vi "GUI.vi"() -> ()   [LabVIEW 2019]
uses:
  <vilib>/Instr/_visa.llb/VISA Configure Serial Port (Instr).vi
panel:
  out "O":dbl
  out "T":dbl
  out "D":dbl
  out "I":dbl
  out "P":dbl
  out "F":dbl
  out "S":dbl
  in  "Stop Button":bool
  out "TS":dbl(slide) scale=0.0..255.0
  out "KD":dbl(slide) scale=0.0..10.0
  out "KI":dbl(slide) scale=0.0..0.1
  out "KP":dbl(slide) scale=0.0..10.0
  in  "COM Port":refnum<visa-resource-name>
  in  "Save Result":path
  out "Output PID":dbl(graph)
  out "Tacho Generator":dbl(knob) scale=0.0..400.0
  out "SetPoint":dbl(knob) scale=0.0..400.0
  out "Respon PID":dynamicdata(graph)
  # "ALIM SATRIA FI'I WIJAYA KUSUMA (21/483503/SV/20304)"
  # "KENDALI KECEPATAN MOTOR DC"
  # "ILHAM DWI CAHYO (21/483417/SV/20218)"
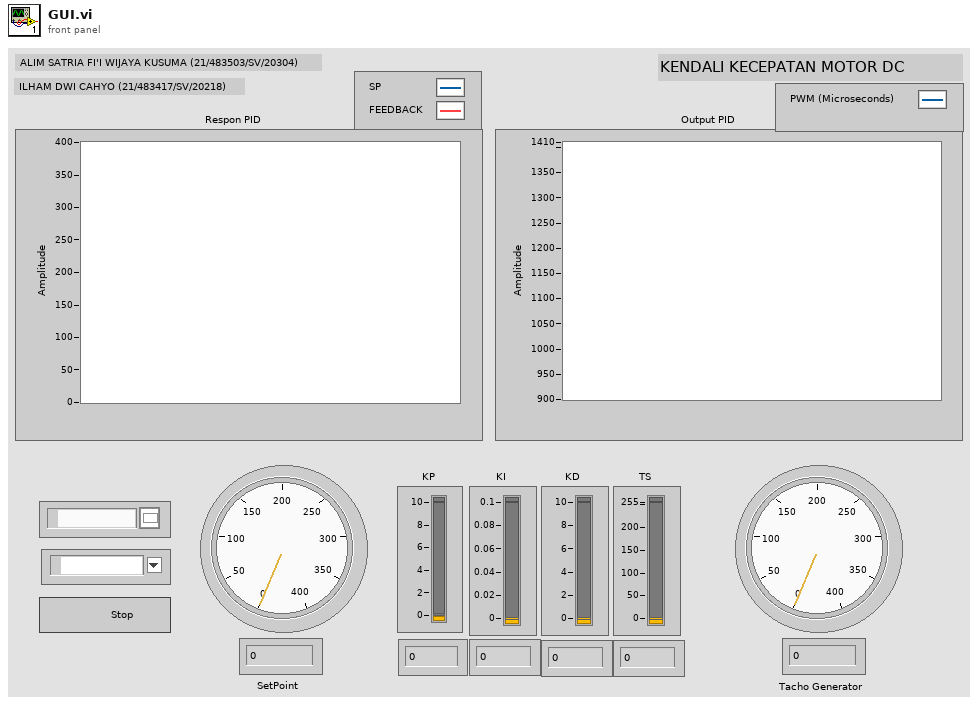
[diagram p1: front panel]
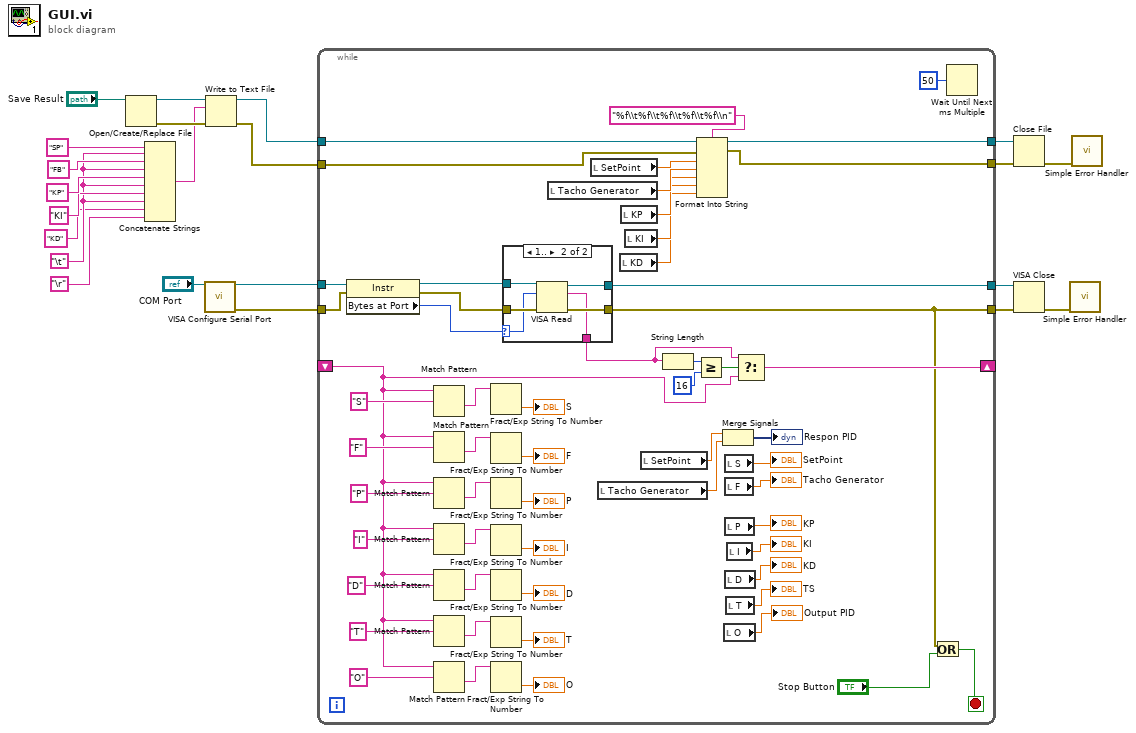
[diagram p0: block diagram]
diagram:
  w5 = "\t"
  n1 = Open/Create/Replace File(file path (use dialog)="Save Result") -> (refnum out=w15:refnum<file>, error out=w16:errorcluster)  [unwired: 5 in, 1 out]
  n2 = Concatenate Strings("SP", w5, "FB" ("string"), w5, "KP" ("string"), w5, "KI" ("string"), w5, "KD" ("string"), "\r") -> (w10:string)
  n3 = call-poly "VISA Configure Serial Port"("VISA resource name"="COM Port") -> ("VISA resource name out"=w22:refnum<visa-resource-name>, "error out"=w21:errorcluster)  [unwired: 13 in]
  n4 = Write to Text File(file (use dialog)=w15, text=w10, error in=w16) -> (refnum out=w14:refnum<file>, error out=w13:errorcluster)  [unwired: 1 in, 1 out]
  n5 = while {
    tunnel: w22 -> [w29]
    tunnel: w21 -> [w24]
    tunnel: [w26] -> w20
    tunnel: [w25] -> w19
    tunnel: w14 -> [w45]
    tunnel: w13 -> [w44]
    tunnel: [w43] -> w12
    tunnel: [w42] -> w11
    shift-right: [w32] -> _
    shift-left: _ -> [w31]
    stop <- w79 stop-if-true
    n6 = property class="Instr"(reference=w29, error in=w24) -> (reference out=w28:refnum<visa-resource-name>, error out=w27:errorcluster, "Bytes at Port"=w77:u32)
    n7 = Match Pattern(string=w31, regular expression="S") -> (after substring=w69:string)  [unwired: 1 in, 3 out]
    n8 = Match Pattern(string=w31, regular expression="F") -> (after substring=w68:string)  [unwired: 1 in, 3 out]
    n9 = Match Pattern(string=w31, regular expression="P") -> (after substring=w67:string)  [unwired: 1 in, 3 out]
    n10 = Match Pattern(string=w31, regular expression="I") -> (after substring=w66:string)  [unwired: 1 in, 3 out]
    n11 = Match Pattern(string=w31, regular expression="D") -> (after substring=w65:string)  [unwired: 1 in, 3 out]
    n12 = Match Pattern(string=w31, regular expression="T") -> (after substring=w64:string)  [unwired: 1 in, 3 out]
    n13 = Match Pattern(string=w31, regular expression="O") -> (after substring=w63:string)  [unwired: 1 in, 3 out]
    n14 = Fract/Exp String To Number(string=w69) -> (number=→"S":dbl)  [unwired: 3 in, 1 out]
    n15 = Fract/Exp String To Number(string=w68) -> (number=→"F":dbl)  [unwired: 3 in, 1 out]
    n16 = Fract/Exp String To Number(string=w67) -> (number=→"P":dbl)  [unwired: 3 in, 1 out]
    n17 = Fract/Exp String To Number(string=w66) -> (number=→"I":dbl)  [unwired: 3 in, 1 out]
    n18 = Fract/Exp String To Number(string=w65) -> (number=→"D":dbl)  [unwired: 3 in, 1 out]
    n19 = Fract/Exp String To Number(string=w64) -> (number=→"T":dbl)  [unwired: 3 in, 1 out]
    n20 = Fract/Exp String To Number(string=w63) -> (number=→"O":dbl)  [unwired: 3 in, 1 out]
    n21 = case shown="1.." w77 {
      selector: w77 -> [_ w82]
      tunnel: w28 -> [w81 w87]
      tunnel: [w81 w86] -> w26
      tunnel: w27 -> [w80 w85]
      tunnel: [w80 w84] -> w25
      tunnel: [_ w83] -> w30
      frame 0, Default {
      }
      frame 1.. {
        n22 = VISA Read(VISA resource name=w87, byte count=w82, error in (no error)=w85) -> (VISA resource name out=w86:refnum<visa-resource-name>, read buffer=w83:string, error out=w84:errorcluster)  [unwired: 1 out]
      }
    }
    n23 = local read "Tacho Generator"() -> (w40:dbl)
    n24 = local read "SetPoint"() -> (w41:dbl)
    n25 = local read "Tacho Generator"() -> (w53:dbl)
    n26 = local read "KD"() -> (w36:dbl)
    n27 = local read "KP"() -> (w38:dbl)
    n28 = local read "KI"() -> (w37:dbl)
    n29 = local read "SetPoint"() -> (w54:dbl)
    n30 = String Length(string=w30) -> (length=w35:i32)
    n31 = Greater Or Equal?(x=w35, y=16) -> (x >= y?=w33:bool)
    n32 = Format Into String(format string="%f\\t%f\\t%f\\t%f\\t%f\\n", initial string=w45, error in=w44, w41, w40, w38, w37, w36) -> (resulting string=w43:refnum<file>, error out=w42:errorcluster)
    n33 = Merge Signals(w54, w53) -> (→"Respon PID":dynamicdata)
    n34 = local read "O"() -> (→"Output PID":dbl)
    n35 = local read "S"() -> (→"SetPoint":dbl)
    n36 = local read "F"() -> (→"Tacho Generator":dbl)
    n37 = local read "P"() -> (→"KP":dbl)
    n38 = local read "D"() -> (→"KD":dbl)
    n39 = local read "T"() -> (→"TS":dbl)
    n40 = local read "I"() -> (→"KI":dbl)
    n41 = Select(t=w30, s=w33, f=w31) -> (s? t:f=w32:string)
    n42 = Or(x=w25, y="Stop Button") -> (x .or. y?=w79:bool)
    n43 = Wait Until Next ms Multiple(millisecond multiple=u32 50) -> ()  [unwired: 1 out]
  }
  n44 = Close File(refnum=w12, error in=w11) -> (error out=w2:errorcluster)  [unwired: 1 out]
  n45 = VISA Close(VISA resource name=w20, error in (no error)=w19) -> (error out=w1:errorcluster)
  n46 = call <vilib>:"Simple Error Handler.vi"("error in (no error)"=w1) -> ()  [unwired: 4 in, 5 out]
  n47 = call <vilib>:"Simple Error Handler.vi"("error in (no error)"=w2) -> ()  [unwired: 4 in, 5 out]
